vi "Spectrum Demo.vi"() -> ()   [LabVIEW 2012]
uses:
  LabVIEW/user.lib/SpectralRadar.llb/set Spectrum Output.vi
  LabVIEW/user.lib/SpectralRadar.llb/display Data 1D.vi
  LabVIEW/user.lib/SpectralRadar.llb/OCT Device.lvclass
  LabVIEW/user.lib/SpectralRadar.llb/Processing.lvclass
  LabVIEW/user.lib/SpectralRadar.llb/Raw Data.lvclass
  LabVIEW/user.lib/SpectralRadar.llb/Data.lvclass
panel:
  in  "stop":bool
  out "Spectrum":dbl[](graph)
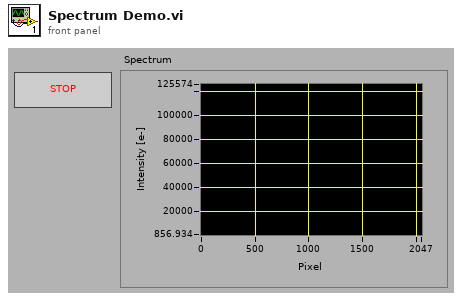
[diagram p1: front panel]
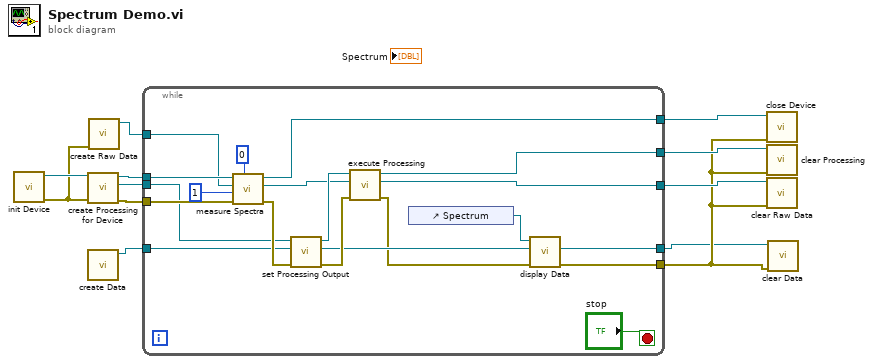
[diagram p0: block diagram]
diagram:
  n1 = call "init Device.vi"() -> ("error out"=w7:errorcluster, "OCTDevice"=w8:refnum<class "OCT Device.lvclass">)  [unwired: 6 in]
  n2 = call "create Processing for Device.vi"("error in (no error)"=w7, "OCTDevice"=w8) -> ("error out"=w9:errorcluster, "Processing"=w11:refnum<class "Processing.lvclass">, "OCTDevice"=w12:refnum<class "OCT Device.lvclass">)  [unwired: 3 in]
  n3 = call "create Data.vi"() -> ("Data"=w3:refnum<class "Data.lvclass">)  [unwired: 6 in, 1 out]
  n4 = call "create Raw Data.vi"("error in (no error)"=w7) -> ("Raw Data"=w10:refnum<class "Raw Data.lvclass">)  [unwired: 5 in, 1 out]
  n5 = while {
    tunnel: w12 -> [w32]
    tunnel: w11 -> [w27]
    tunnel: w10 -> [w31]
    tunnel: w9 -> [w29]
    tunnel: [w20] -> w4
    tunnel: [w19] -> w5
    tunnel: [w18] -> w1
    tunnel: [w17] -> w6
    tunnel: [w16] -> w2
    tunnel: w3 -> [w14]
    stop <- "stop" stop-if-true
    n6 = call "measure Spectra.vi"("Camera #"=0, "error in (no error)"=w29, "NumberOfSpectra"=1, "Raw Data"=w31, "OCTDevice"=w32) -> ("error out"=w28:errorcluster, "Raw Data"=w25:refnum<class "Raw Data.lvclass">, "OCTDevice"=w17:refnum<class "OCT Device.lvclass">)  [unwired: 1 in]
    n7 = call-poly "set Processing Output.vi"("error in (no error)"=w28, "Data"=w14, "Processing"=w27) -> ("error out"=w24:errorcluster, "Data"=w23:refnum<class "Data.lvclass">, "Processing"=w26:refnum<class "Processing.lvclass">)  [unwired: 2 in]
    n8 = call "execute Processing.vi"("error in (no error)"=w24, "Raw Data"=w25, "Processing"=w26) -> ("error out"=w21:errorcluster, "Raw Data"=w20:refnum<class "Raw Data.lvclass">, "Processing"=w19:refnum<class "Processing.lvclass">)  [unwired: 2 in]
    n9 = control-ref of="Spectrum"() -> (w22:refnum<vi>)
    n10 = call-poly "display Data.vi"("error in (no error)"=w21, "Data in"=w23, "WFGraph Refnum"=w22) -> ("error out"=w16:errorcluster, "Data out"=w18:refnum<class "Data.lvclass">)  [unwired: 2 in, 1 out]
  }
  n11 = call "close Device.vi"("error in (no error)"=w2, "OCTDevice"=w6) -> ()  [unwired: 5 in, 1 out]
  n12 = call "clear Processing.vi"("error in (no error)"=w2, "Processing"=w5) -> ()  [unwired: 5 in, 1 out]
  n13 = call "clear Raw Data.vi"("error in (no error)"=w2, "Raw Data"=w4) -> ()  [unwired: 5 in, 1 out]
  n14 = call "clear Data.vi"("error in (no error)"=w2, "Data"=w1) -> ()  [unwired: 5 in, 1 out]
